vi "Create New Record.vi"(6 "Serializer":refnum<class "Serializer.lvclass">, 7 "Record in":refnum<class "Record.lvclass">, 8 "error in (no error)":errorcluster, 10 "Message":string, 11 "Level":T1(ring)) -> (0 "error out":errorcluster, 3 "Record out":refnum<class "Record.lvclass">)   [LabVIEW 2017, in "Error Log.lvlib" / "Record.lvclass"]
uses:
  Record.lvclass
  Serializer/Serializer.lvclass
  Record.lvclass/Record.ctl
  Set Level.vi
  Set Message.vi
  Set Time Stamp.vi
  Set Serializer.vi
  timeStampToString.vi
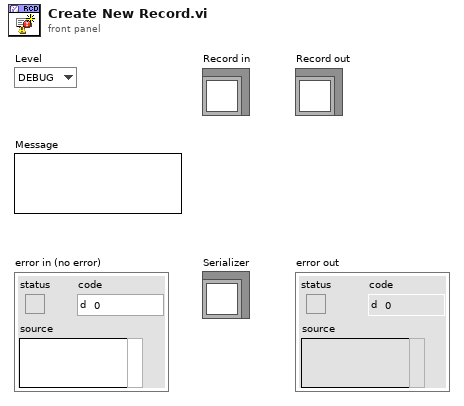
[diagram p1: front panel]
types:
  T1 = enum16{"DEBUG", "INFO", "WARNING", "ERROR", "CRITICAL"}
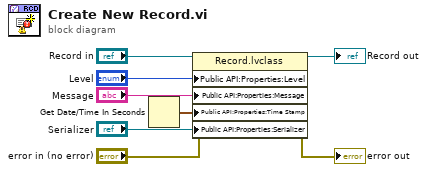
[diagram p0: block diagram]
diagram:
  n1 = Get Date/Time In Seconds() -> (seconds since 1Jan1904=w5:timestamp)
  n2 = property class="Record.lvclass"(reference="Record in", error in="error in (no error)", "Public API:Properties:Level"="Level", "Public API:Properties:Message"="Message", "Public API:Properties:Time Stamp"=w5, "Public API:Properties:Serializer"="Serializer") -> (reference out=→"Record out":refnum<class "Record.lvclass">, error out=→"error out":errorcluster)
